vi "create default alias.vi"(8 "error in":errorcluster, 11 "configuration in":refnum<class "sbRIO-9651 Configuration.lvclass">) -> (0 "error out":errorcluster, 2 "default alias":string, 3 "configuration out":refnum<class "sbRIO-9651 Configuration.lvclass">)   [LabVIEW 2014, in "sbRIO-9651 Configuration.lvclass"]
uses:
  sbRIO-9651 Configuration.lvclass
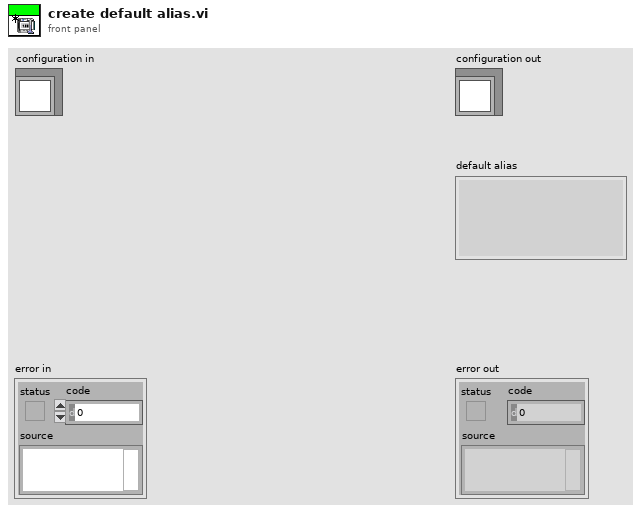
[diagram p1: front panel]
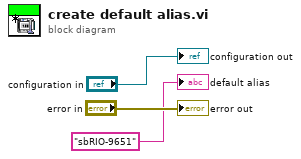
[diagram p0: block diagram]
diagram:
  "error out" <- "error in"
  "configuration out" <- "configuration in"
  "default alias" <- "sbRIO-9651" ("text")
